vi "5p1_HW_Task1_gamagetd.vi"() -> ()   [LabVIEW 2016]
panel:
  out "Electrostatic Force":dbl
  out "Attract, repel or neither":string
  in  "Distance in meters":dbl
  in  "Q2":dbl
  in  "Q1":dbl
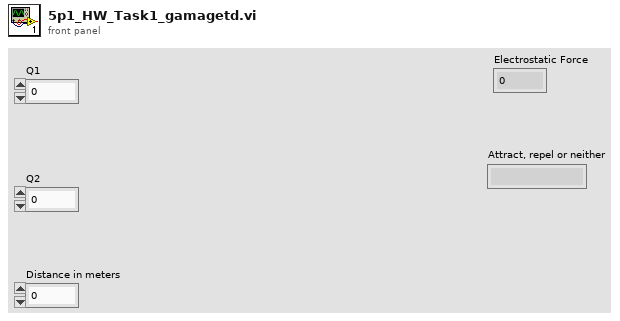
[diagram p1: front panel]
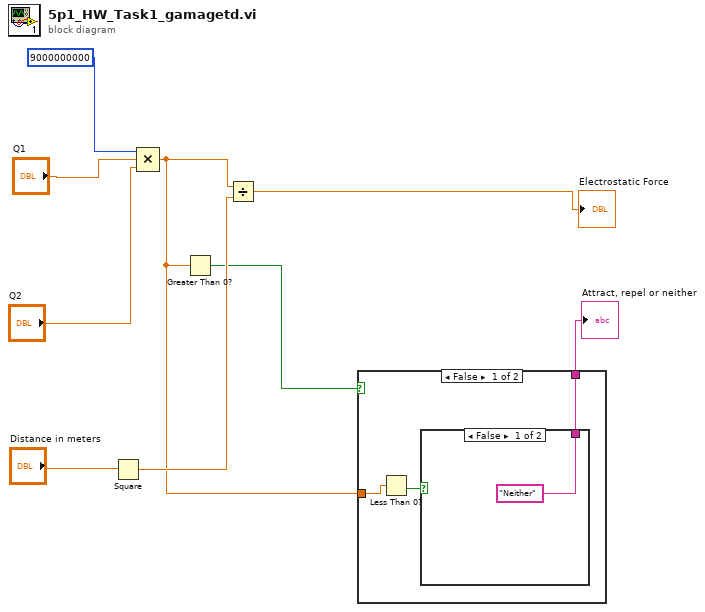
[diagram p0: block diagram]
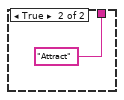
[diagram p2: hidden frame]
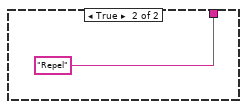
[diagram p3: hidden frame]
diagram:
  n1 = Square(x="Distance in meters") -> (x^2=w5:dbl)
  n2 = Compound Arithmetic op=MULTIPLY(i64 9000000000, "Q1", "Q2") -> (w2:dbl)
  n3 = Greater Than 0?(x=w2) -> (x > 0?=w3:bool)
  n4 = Divide(x=w2, y=w5) -> (x/y=→"Electrostatic Force":dbl)
  n5 = case shown="False" w3 {
    tunnel: w2 -> [w10 _]
    tunnel: [w12 "Repel"] -> w1
    frame False {
      n6 = Less Than 0?(x=w10) -> (x < 0?=w11:bool)
      n7 = case shown="False" w11 {
        tunnel: ["Neither" "Attract"] -> w12
        frame False {
        }
        frame True {
        }
      }
    }
    frame True {
    }
  }
  "Attract, repel or neither" <- w1
